vi "RT Driver VI.vi"(0 "Sensor Model":T1, 1 "bitfile address":path, 2 "ambient T, sensor t0, and heat params":dbl[](array[numeric]), 3 "RIO address":string, 5 "thermal model rate":dbl, 9 "Device Inputs FIFO":refnum<k33>, 10 "Device Outputs FIFO":refnum<k33>, 11 "Device Reference":T2 format="%.0x") -> ()   [LabVIEW 2014, in "UEGO Sim Engine.lvlib"]
uses:
  UEGO Sim Engine.lvlib
  <vilib>/NI Veristand/Custom Device API/Custom Device Item Ref.ctl
  <vilib>/NI Veristand/Custom Device API/Custom Device Channel Type.ctl
  UEGO CD state.ctl
  Shared/UEGO fpga inputs.ctl
  Shared/UEGO fpga outputs.ctl
  Shared/VS input channels.ctl
  Shared/VS output channels.ctl
  Shared/Constants.vi
  <vilib>/FPGAPlugInAG/Dynamic/niLvFpga_Close_Dynamic.vi
  <vilib>/rvi/interface/nirviCloseFPGA/nirviCloseFPGA.xnode
  <vilib>/NI Veristand/Custom Device API/Custom Device API.lvlib
  <vilib>/NI Veristand/Custom Device Tools/Custom Device Utility Library/Custom Device Utility Library.lvlib
  Shared/UEGO Sim Shared.lvlib
panel:
  in  "Initialization Status Notifier":refnum<notifier>
  in  "Status Notifier":refnum<notifier>
  # "Custom Device Template\nv1.0"
  # "Use this template as a starting point for creating a custom device code module. The input controls shown here are specially named controls that the system will use to provide the device loop with data. The controls are not required for the device loop to run. For instance, if the device doesn't produce any output data, then you don't need the Device Outputs FIFO control. If you do use these controls, however, they need to have these exact names to be functional."
  # "The optional status notifier element is used to notify the RT engine of the last state of the custom device, and to indicate the device has completed execution. If this control is not used, a default No Error value is returned to the system when the device finishes execution.\n\nNote: This error state is not checked until the system shuts down. Use an output status channel to send more immediate status values to the system."
  # "This optional input can be used to send the VeriStand Engine the final status of the custom device initalization process. If this control exists on the custom device front panel, the VeriStand Engine will wait for a status update before starting up. If the custom device reports an error, that will abort the execution of the current configuration in the VeriStand Engine.\n\nThis control can be deleted if the custom device does not need to send the initialization status update."
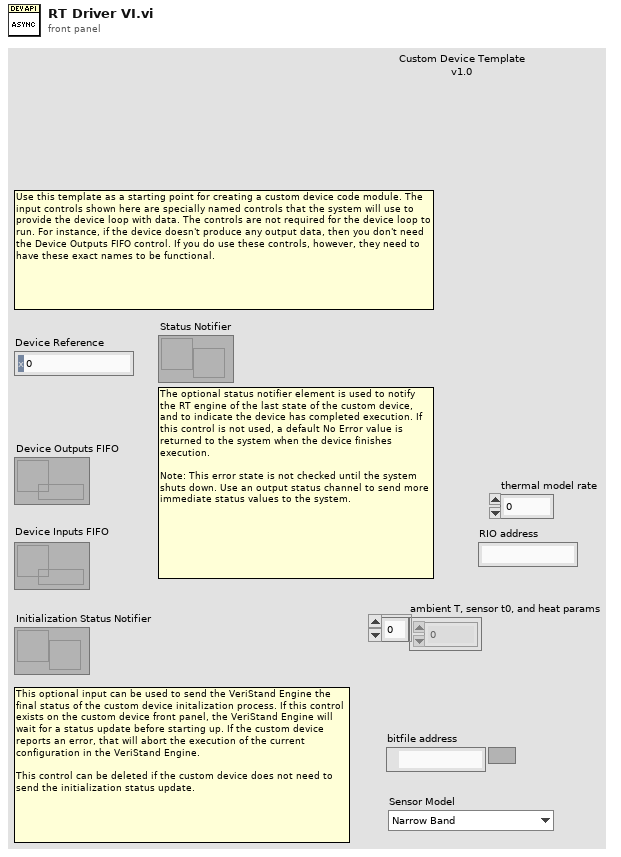
[diagram p1: front panel]
types:
  T1 = typedef "UEGO Sim Shared.lvlib/sensor models" = enum16{"Narrow Band", "Bosch 4.2", "Bosch 4.9"}
  T2 = typedef "Custom Device API.lvlib/Custom Device Item Ref.ctl" = u64
  T3 = typedef "Custom Device API.lvlib/Custom Device Channel Type.ctl" = enum16{"Input", "Output"}
  T4 = typedef "UEGO Sim Engine.lvlib/UEGO CD state.ctl" = cluster{"FPGA in":T5, "FPGA out":T6, "FPGA in ref":refnum<k20>, "FPGA out ref":refnum<k20>, "VS input channels":T7, "VS output channels":T8, "FPGA cal input ref":refnum<k20>, "FPGA cal offset ref":refnum<k20>}
  T5 = typedef "UEGO Sim Shared.lvlib/UEGO fpga inputs.ctl" = cluster{"PWM low time":u32, "PWM high time":u32}
  T6 = typedef "UEGO Sim Shared.lvlib/UEGO fpga outputs.ctl" = cluster{"Sensor Model":T1, "lambda":fxp<+,12,3>, "cal":bool, "negate":bool, "PWM threshold":i16, "PWM timeout":u32}
  T7 = typedef "UEGO Sim Shared.lvlib/VS input channels.ctl" = cluster{"lambda":dbl, "thermal reset":dbl, "PWM timeout":dbl, "PWM threshold":dbl, "Heater Invert":dbl, "Calibrate":dbl}
  T8 = typedef "UEGO Sim Shared.lvlib/VS output channels.ctl" = cluster{"resistance out":dbl, "temp out":dbl, "heater duty cycle out":dbl}
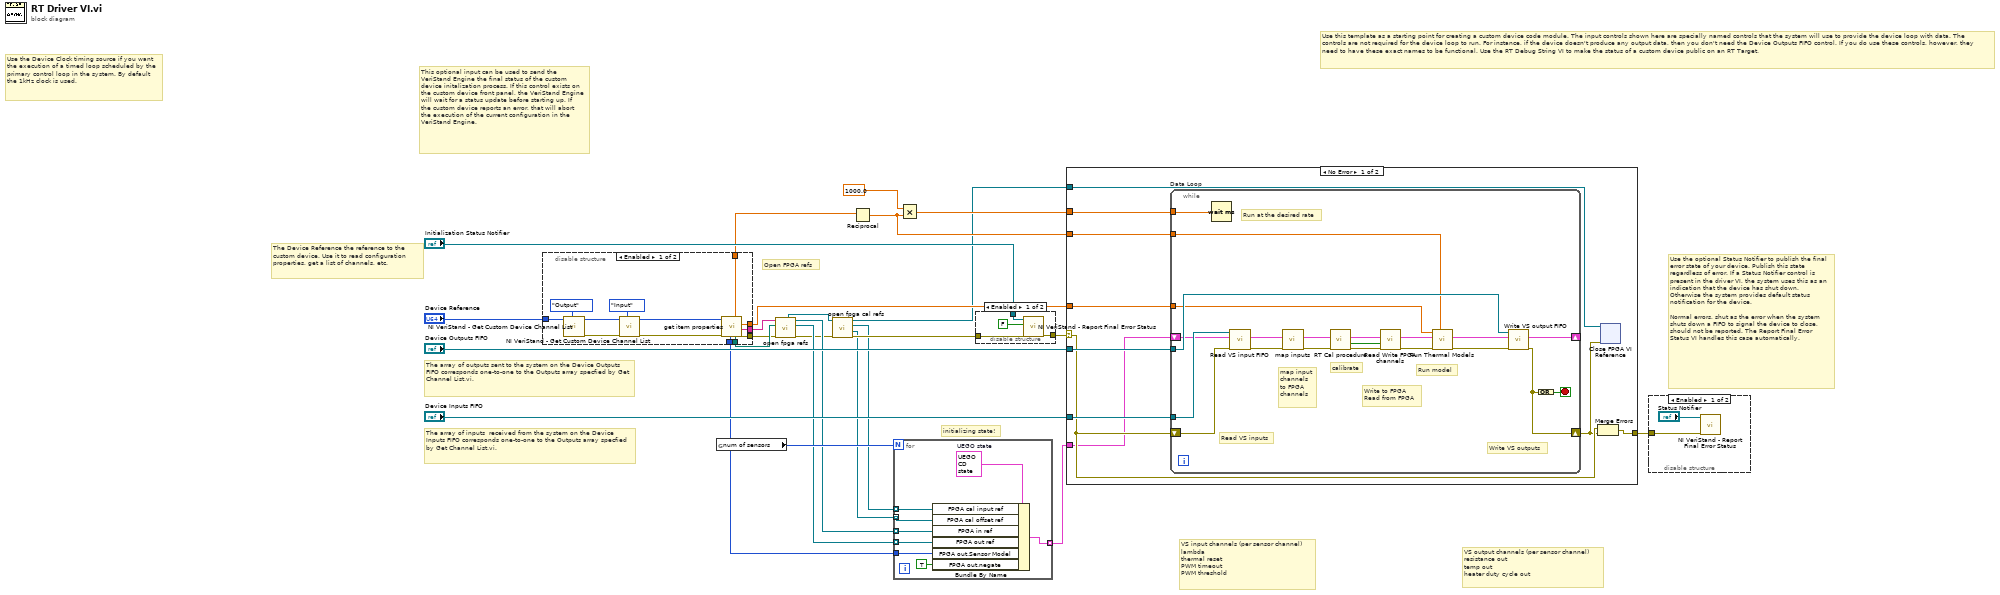
[diagram p0: block diagram]
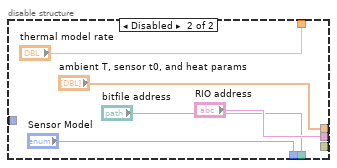
[diagram p4: hidden frame]
diagram:
  # "initializing state!"
  # "VS output channels (per sensor channel)\nresistance out\ntemp out\nheater duty cycle out"
  # "VS input channels (per sensor channel)\nlambda \nthermal reset\nPWM timeout\nPWM threshold"
  # "Open FPGA refs"
  # "This optional input can be used to send the VeriStand Engine the final status of the custom device initalization process. If this control exists on the custom device front panel, the VeriStand Engine will wait for a status update before starting up. If the custom device reports an error, that will abort the execution of the current configuration in the VeriStand Engine."
  # "The array of inputs  received from the system on the Device Inputs FIFO corresponds one-to-one to the Outputs array specfied by Get Channel List.vi."
  # "Use the optional Status Notifier to publish the final error state of your device. Publish this state regardless of error. If a Status Notifier control is present in the driver VI, the system uses this as an indication that the device has shut down. Otherwise the system provides default status notification for the device.\n\nNormal errors, shut as the error when the system shuts down a FIFO to signal the device to close, should not be reported. The Report Final Error Status VI handles this case automatically."
  # "The array of outputs sent to the system on the Device Outputs FIFO corresponds one-to-one to the Outputs array specfied by Get Channel List.vi."
  # "The Device Reference the reference to the custom device. Use it to read configuration properties, get a list of channels, etc."
  # "Use the Device Clock timing source if you want the execution of a timed loop scheduled by the primary control loop in the system. By default the 1kHz clock is used."
  # "Use this template as a starting point for creating a custom device code module. The input controls shown here are specially named controls that the system will use to provide the device loop with data. The controls are not required for the device loop to run. For instance, if the device doesn't produce any output data, then you don't need the Device Outputs FIFO control. If you do use these controls, however, they need to have these exact names to be functional. Use the RT Debug String VI to make the status of a custom device public on an RT Target."
  n1 = disable-structure shown="Enabled" {
    disable-tunnel: "Device Reference" -> [w34 _]
    disable-tunnel: [w31 "ambient T, sensor t0, and heat params"] -> w19
    disable-tunnel: [w30 "RIO address"] -> w16
    disable-tunnel: [w29 "bitfile address"] -> w15
    disable-tunnel: [w28 _] -> w14
    disable-tunnel: [w27 "Sensor Model"] -> w13
    disable-tunnel: [w26 "thermal model rate"] -> w10
    frame Enabled {
      n2 = call <vilib>:"NI VeriStand - Get Custom Device Channel List.vi"("Channel Type"=Custom_Device_Channel_Type."Output", "Device Ref in"=w34) -> ("error out"=w36:errorcluster, "Device Ref out"=w37:T2)  [unwired: 1 in, 7 out]
      n3 = call <vilib>:"NI VeriStand - Get Custom Device Channel List.vi"("Channel Type"=Custom_Device_Channel_Type."Input", "error in (no error)"=w36, "Device Ref in"=w37) -> ("error out"=w32:errorcluster, "Device Ref out"=w33:T2)  [unwired: 7 out]
      n4 = call "get item properties.vi"("error in (no error)"=w32, "Device Ref in"=w33) -> ("error out"=w28:errorcluster, "RIO target"=w30:string, "ambient T, sensor t0, and heat params"=w31:dbl[], "Path"=w29:path, "thermal model rate"=w26:dbl, "Sensor Model"=w27:T1)  [unwired: 4 in]
    }
    frame Disabled {
    }
  }
  n5 = global read "Constants.vi" "num of sensors"() -> (w11:i32)
  n6 = call "open fpga refs.vi"("error in (no error)"=w14, "bitfile address"=w15, "RIO address"=w16) -> ("error out"=w4:errorcluster, "FPGA out refs"=w7:refnum<k20>[], "FPGA in refs"=w8:refnum<k20>[], "Top level fpga ref"=w6:refnum<k20>)  [unwired: 5 in]
  n7 = call "open fpga cal refs.vi"("Error In"=w4, "Top level fpga ref"=w6) -> ("Error out"=w3:errorcluster, "Cal offset refs"=w2:refnum<k20>[], "Cal input refs"=w1:refnum<k20>[], "Top level fpga ref"=w5:refnum<k20>)  [unwired: 6 in]
  n8 = Reciprocal(x=w10) -> (1/x=w9:dbl)
  n9 = for {
    N: w11 -> [_]
    tunnel: w8 -> [w51] mode=indexing
    tunnel: w7 -> [w50] mode=indexing
    tunnel: w13 -> [w49]
    tunnel: [w48] -> w12 mode=indexing
    tunnel: w2 -> [w45] mode=indexing
    tunnel: w1 -> [w44] mode=indexing
    w47 = T4 {"FPGA in"={"PWM low time"=0, "PWM high time"=0}, "FPGA out"={"Sensor Model"=enum."Narrow Band", "lambda"=1.0, "cal"=FALSE, "negate"=FALSE, "PWM threshold"=1500, "PWM timeout"=40000}, "FPGA in ref"=refnum, "FPGA out ref"=refnum, "VS input channels"={"lambda"=0.0, "thermal reset"=0.0, "PWM timeout"=0.0, "PWM threshold"=0.0, "Heater Invert"=0.0, "Calibrate"=0.0}, "VS output channels"={"resistance out"=0.0, "temp out"=0.0, "heater duty cycle out"=0.0}, "FPGA cal input ref"=refnum, "FPGA cal offset ref"=refnum}  # UEGO state
    n10 = Bundle By Name(cluster=w47, "FPGA cal input ref"=w44, "FPGA cal offset ref"=w45, "FPGA in ref"=w51, "FPGA out ref"=w50, "FPGA out.Sensor Model"=w49, "FPGA out.negate"=TRUE) -> (w48:T4)
  }
  n11 = Multiply(x=1000.0, y=w9) -> (x*y=w17:dbl)
  n12 = disable-structure shown="Enabled" {
    disable-tunnel: "Initialization Status Notifier" -> [w55 _]
    disable-tunnel: [w54 w56] -> w20
    disable-tunnel: w3 -> [w52 w56]
    frame Enabled {
      n13 = call <vilib>:"NI VeriStand - Report Final Error Status.vi"("error in (no error)"=w52, "Filter FIFO & Shutdown Errors (T)"=FALSE ("Filter FIFO Errors (T)"), "Status Notifier"=w55) -> ("error out"=w54:errorcluster)  [unwired: 8 out]
    }
    frame Disabled {
    }
  }
  n14 = case shown="No Error" w20 {
    selector: w20 -> [w64 w88]
    tunnel: "Device Outputs FIFO" -> [w66 _]
    tunnel: "Device Inputs FIFO" -> [w65 _]
    tunnel: [w63 w88] -> w22
    tunnel: w19 -> [w60 _]
    tunnel: w17 -> [w62 _]
    tunnel: w12 -> [w61 _]
    tunnel: w9 -> [w59 _]
    tunnel: w5 -> [w57 _]
    frame No Error {
      n15 = while "Data Loop" {
        shift-right: [w82] -> w58
        shift-left: w64 -> [w84]
        tunnel: w66 -> [w83]
        tunnel: w65 -> [w85]
        tunnel: w62 -> [w86]
        shift-right: [w75] -> _
        shift-left: w61 -> [w74]
        tunnel: w60 -> [w80]
        tunnel: w59 -> [w79]
        stop <- w87 stop-if-true
        # "calibrate"
        # "Run model"
        # "Write to FPGA\nRead from FPGA"
        # "map input\nchannels\nto FPGA\nchannels"
        # "Write VS outputs"
        # "Read VS inputs"
        # "Run at the desired rate"
        n16 = Wait (ms)(milliseconds to wait=w86) -> ()  [unwired: 1 out]
        n17 = call "Read VS input FIFO.vi"("error in (no error)"=w84, "CD state in"=w74, "Refnum in"=w85) -> ("error out (no error)"=w77:errorcluster, "CD state out"=w81:T4[])  [unwired: 7 in]
        n18 = call "map inputs.vi"("Error In"=w77, "CD state in"=w81) -> ("Error Out"=w71:errorcluster, "CD state out"=w69:T4[])  [unwired: 8 in]
        n19 = call "RT Cal procedure.vi"("Error In"=w71, "CD State in"=w69) -> ("error out"=w70:errorcluster, "Channels in Cal mode?"=w67:bool[], "CD State out"=w68:T4[])  [unwired: 7 in]
        n20 = call "Read Write FPGA channels.vi"("error in"=w70, "Channels in Cal mode?"=w67, "CD state in"=w68) -> ("error out"=w72:errorcluster, "CD state out"=w73:T4[])  [unwired: 7 in]
        n21 = call "Run Thermal Models.vi"("thermal dt"=w79, "Error In"=w72, "CD state in"=w73, "ambient T, sensor t0, and heat params"=w80) -> ("Error Out"=w76:errorcluster, "CD  state out"=w78:T4[])  [unwired: 6 in]
        n22 = call "Write VS output FIFO.vi"("error in (no error)"=w76, "CD  state in"=w78, "Refnum in"=w83) -> ("error out"=w82:errorcluster, "CD State out"=w75:T4[])  [unwired: 7 in]
        n23 = Compound Arithmetic op=OR(w82) -> (w87:bool)
      }
      n24 = Merge Errors(w64, w58) -> (w63:errorcluster)
      n25 = xnode "Close FPGA VI Reference"("FPGA VI Reference In"=w57, "error in"=w58) -> ()  [unwired: 1 out]
    }
    frame Error {
    }
  }
  n26 = disable-structure shown="Enabled" {
    disable-tunnel: w22 -> [w89 _]
    frame Enabled {
      n27 = call <vilib>:"NI VeriStand - Report Final Error Status.vi"("error in (no error)"=w89, "Status Notifier"="Status Notifier") -> ()  [unwired: 1 in, 9 out]
    }
    frame Disabled {
    }
  }
